vi "Edit PWM Output.vi"(8 "error in":errorcluster, 10 "PWM Data in":T1={"Frequency"=1000.0, "Duty Cycle"=0.5, "PWM Action"=enum."PWM Start"}, 11 "Sequence Context In":refnum<k7>) -> (0 "error out":errorcluster, 2 "PWM Data out":T1={"Frequency"=1000.0, "Duty Cycle"=0.99, "PWM Action"=enum."PWM Start"})   [LabVIEW 2023, in "LTT_TeststandSteptypes.lvlib"]
uses:
  LTT_TeststandSteptypes.lvlib
  Control/PWM Output Data.ctl
  <vilib>/addons/TestStand/_TSUtility.llb/TestStand - Start Modal Dialog (Sequence Context).vi
  <vilib>/addons/TestStand/_TSUtility.llb/TestStand - End Modal Dialog (Sequence Context).vi
panel:
  in  "Close":bool
  in  "OK":bool
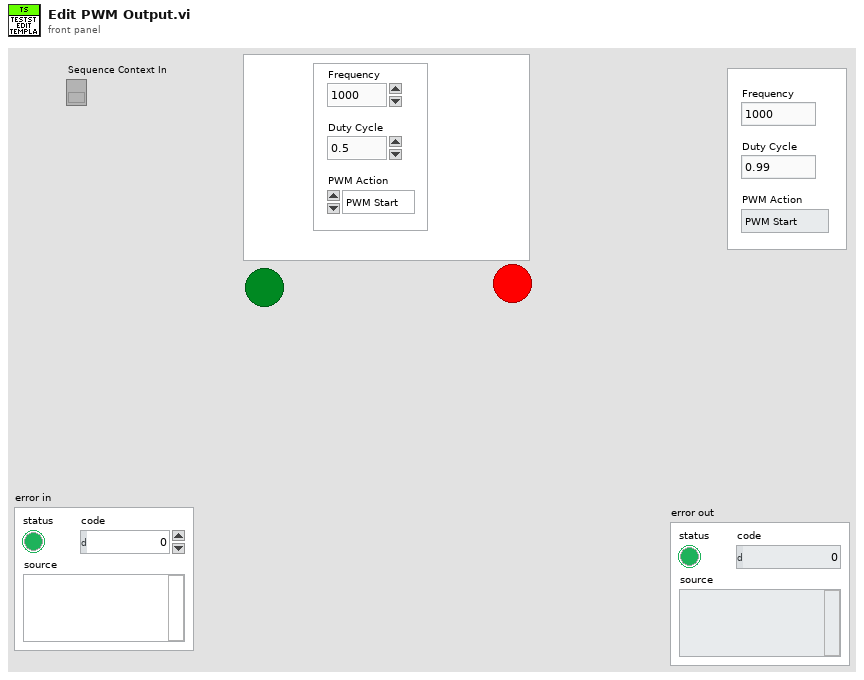
[diagram p1: front panel]
types:
  T1 = typedef "LTT_TeststandSteptypes.lvlib/PWM Output Data.ctl" = cluster{"Frequency":dbl, "Duty Cycle":dbl, "PWM Action":enum16{"PWM Start", "PWM Stop"}}
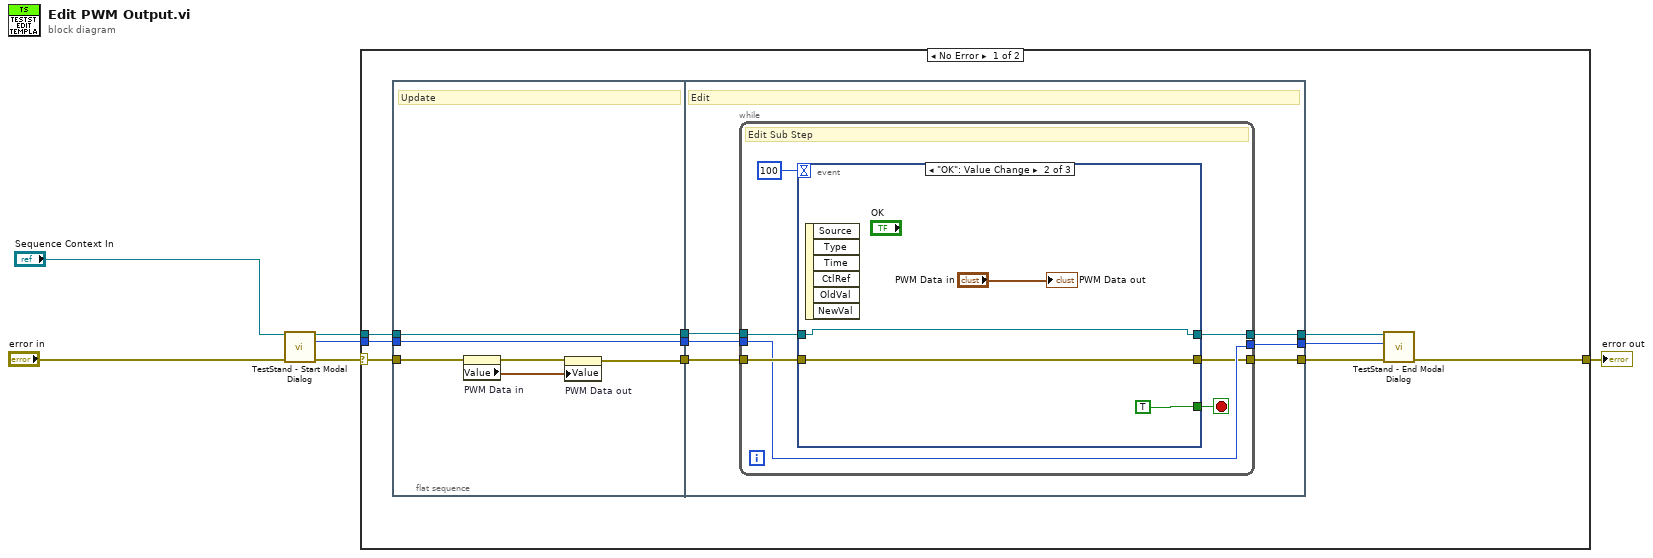
[diagram p0: block diagram]
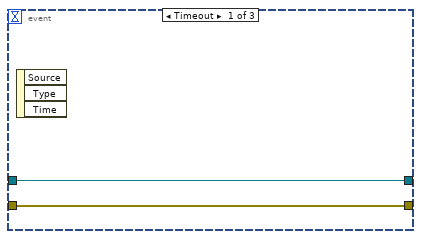
[diagram p2: hidden frame]
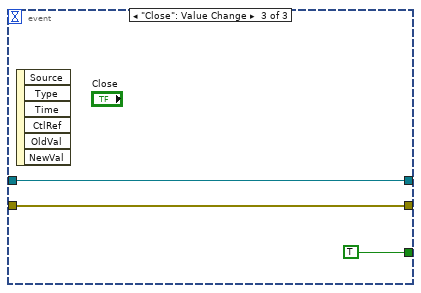
[diagram p3: hidden frame]
diagram:
  n1 = call-poly <vilib>:"TestStand - Start Modal Dialog.vi"("Sequence Context In"="Sequence Context In", "error in (no error)"="error in") -> ("Sequence Context Out"=w4:refnum<k7>, "Modal ID"=w3:i32, "error out"=w5:errorcluster)  [unwired: 9 in, 2 out]
  n2 = case shown="No Error" w5 {
    selector: w5 -> [w13 w45]
    tunnel: w4 -> [w10 _]
    tunnel: w3 -> [w9 _]
    tunnel: [w11 w45] -> w1
    frame No Error {
      n3 = flat-sequence {
        tunnel: w13 -> [w20]
        tunnel: [w18] -> w16
        tunnel: w10 -> [w22]
        tunnel: w9 -> [w21]
        tunnel: [w22] -> w15
        tunnel: [w21] -> w14
        tunnel: w16 -> [w26]
        tunnel: [w24] -> w12
        tunnel: w15 -> [w28]
        tunnel: w14 -> [w27]
        tunnel: [w25] -> w8
        tunnel: [w23] -> w7
        frame #0 {
          # "Update"
          n4 = property on="PWM Data in" class="Clust (strict)"(error in=w20) -> (error out=w19:errorcluster, "Value"=w17:T1)  [unwired: 1 in, 1 out]
          n5 = property on="PWM Data out" class="Clust (strict)"(error in=w19, "Value"=w17) -> (error out=w18:errorcluster)  [unwired: 1 in, 1 out]
        }
        frame #1 {
          # "Edit"
          n6 = while {
            tunnel: w28 -> [w33]
            tunnel: w27 -> [w30]
            tunnel: w26 -> [w31]
            tunnel: [w32] -> w23
            tunnel: [w30] -> w25
            tunnel: [w29] -> w24
            stop <- w34 stop-if-true
            # "Edit Sub Step"
            n7 = event shown="[1] \"OK\": Value Change" {
              selector: _ -> [_ _ _]
              dyn-events: _ -> [_ _ _]
              timeout: 100 -> [_ _ _]
              tunnel: [_ TRUE TRUE] -> w34
              tunnel: [w37 w38 w43] -> w32
              tunnel: w33 -> [w37 w38 w43]
              tunnel: w31 -> [w36 w39 w42]
              tunnel: [w36 w39 w42] -> w29
              event Timeout {
                n8 = event-data() -> ()  [unwired: 1 in, 3 out]
              }
              event "OK": Value Change {
                n9 = event-data() -> ()  [unwired: 1 in, 6 out]
                "PWM Data out" <- "PWM Data in"
              }
              event "Close": Value Change {
                n10 = event-data() -> ()  [unwired: 1 in, 6 out]
              }
            }
          }
        }
      }
      n11 = call-poly <vilib>:"TestStand - End Modal Dialog.vi"("Sequence Context In"=w7, "Modal ID"=w8, "error in (no error)"=w12) -> ("error out"=w11:errorcluster)  [unwired: 12 in]
    }
    frame Error {
    }
  }
  "error out" <- w1
